vi "Test Hermitian (CDB).vi"(9 "relative tolerance?":bool, 10 "tolerance":dbl=-1.0, 11 "Input Matrix":T1) -> (0 "error":i32, 3 "Hermitian?":bool)   [LabVIEW 2018, in "NI_AALPro.lvlib"]
uses:
  NI_AALPro.lvlib
  ComplexMatrix.ctl
  <resource>/lvanlys.dll
  NI_Matrix.lvlib
panel:
  # "Test Hermitian"
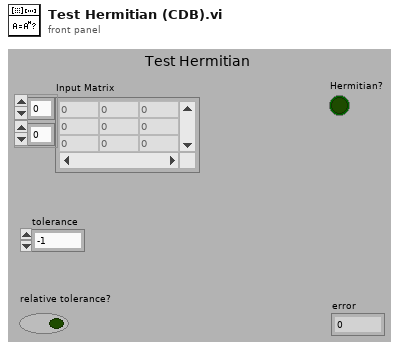
[diagram p1: front panel]
types:
  T1 = typedef "NI_Matrix.lvlib/ComplexMatrix.ctl" = cdb[][]
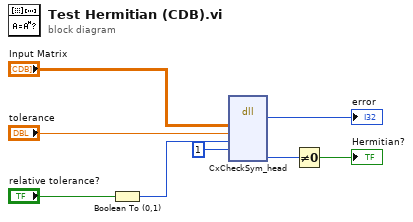
[diagram p0: block diagram]
diagram:
  n1 = Boolean To (0,1)(Boolean="relative tolerance?") -> (0, 1=w5:i16)
  n2 = dll-call lib="C:/Program Files (x86)/National Instruments/LabVIEW 2018/resource/lvanlys.*" fn="CxCheckSym_head" ("lvanlys.dll:CxCheckPosSemiDef_head")("_aH"="Input Matrix", "_tol"="tolerance", "_reltol"=w5, "_conj"=1) -> ("return type"=→"error":i32, "_sym"=w4:i32)  [unwired: 6 in, 4 out]
  n3 = Not Equal To 0?(x=w4) -> (x != 0?=→"Hermitian?":bool)
